vi "SYST_ACT_CHAN.vi"(0 "VISA IN":refnum<visa-resource-name>, 5 "error in":errorcluster) -> (13 "Channel":i32, 14 "VISA Out":refnum<visa-resource-name>, 19 "error out":errorcluster)   [LabVIEW 2018, in "PNA-X.lvlib"]
doc: "SYSTem:ACTive:CHANnel? \n(Read-only) Returns the number of the active channel or an error message if there is no active \nchannel. The active channel is the channel number that contains the active measurement. \nExamples SYST:PRES \nSYST:ACT:CHAN? \n'Returns 1 \nReturn Type Integer \nDefault Not Applicable"
uses:
  PNA-X.lvlib
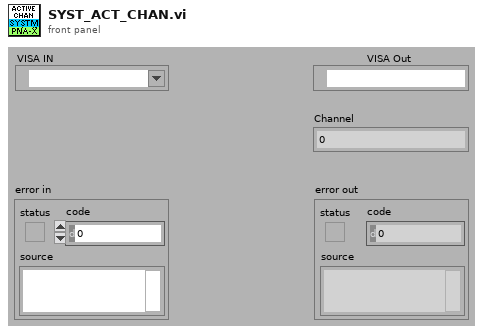
[diagram p1: front panel]
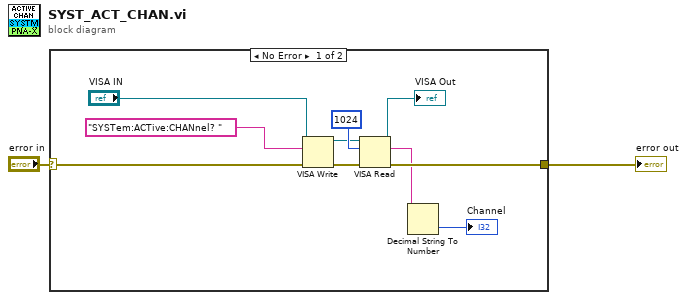
[diagram p0: block diagram]
diagram:
  n1 = case shown="No Error" "error in" {
    selector: "error in" -> [w6 w13]
    tunnel: [w8 w13] -> w1
    frame No Error {
      n2 = VISA Write(VISA resource name="VISA IN", write buffer="SYSTem:ACTive:CHANnel? " ("Cmdline"), error in (no error)=w6) -> (VISA resource name out=w9:refnum<visa-resource-name>, error out=w11:errorcluster)  [unwired: 1 out]
      n3 = VISA Read(VISA resource name=w9, byte count=1024, error in (no error)=w11) -> (VISA resource name out=→"VISA Out":refnum<visa-resource-name>, read buffer=w4:string, error out=w8:errorcluster)  [unwired: 1 out]
      n4 = Decimal String To Number(string=w4) -> (number=→"Channel":i32)  [unwired: 2 in, 1 out]
    }
    frame Error {
    }
  }
  "error out" <- w1
